vi "Retry Num.vi"(11 "String":string) -> (2 "Numeric":i32, 3 "retryΩ计":string[](array[string]))   [LabVIEW 2019, in "LineScan.lvclass"]
uses:
  LineScan/LineScan.lvclass
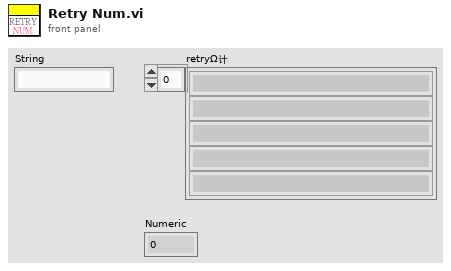
[diagram p1: front panel]
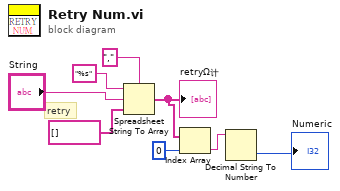
[diagram p0: block diagram]
diagram:
  # "retry"
  n1 = Spreadsheet String To Array(delimiter (Tab)=",", format string="%s", spreadsheet string="String", array type (2D Dbl)=string[] []) -> (array=w5:string[])
  "retryΩ计" <- w5
  n2 = Index Array(array=w5, index=0) -> (element=w7:string)
  n3 = Decimal String To Number(string=w7) -> (number=→"Numeric":i32)  [unwired: 2 in, 1 out]
